vi "Launch Rectangular Mask.vi"(4 "Color":u32, 6 "Transparency":u8, 9 "Monitor":i32, 10 "Bounds":T2) -> (2 "Panels (cluster)":T1, 3 "Panels (array)":refnum<vi>[](array[refnum]))   [LabVIEW 2016, in "Rectangle Mask.lvclass"]
uses:
  Classes/Rectangle Mask/Rectangle Mask.lvclass
  <vilib>/Utility/miscctls.llb/LVRectTypeDef.ctl
  Classes/Rectangle Mask/Panels.ctl
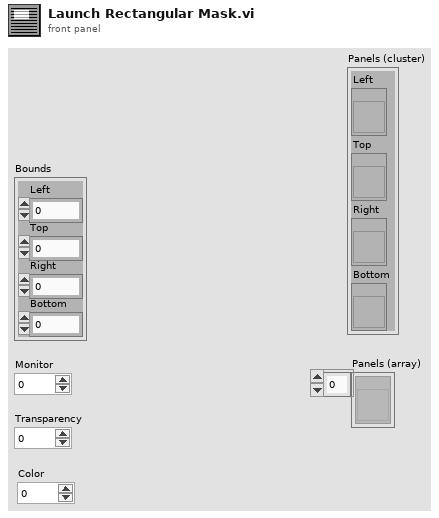
[diagram p1: front panel]
types:
  T1 = typedef "Rectangle Mask.lvclass/Panels.ctl" = cluster{"Left":refnum<vi>, "Top":refnum<vi>, "Right":refnum<vi>, "Bottom":refnum<vi>}
  T2 = typedef "LVRectTypeDef.ctl" = cluster{"Left":i16, "Top":i16, "Right":i16, "Bottom":i16}
  T3 = enum32{"Invalid", "Standard", "Closed", "Hidden", "Minimized", "Maximized"}
  T4 = typedef "LVAllMonitorsDisplayTypeDef.ctl" = cluster{"Bounds":cluster{"Left":i16, "Top":i16, "Right":i16, "Bottom":i16}, "Depth":i16}[]
  T5 = cluster{"Bounds":cluster{"Left":i16, "Top":i16, "Right":i16, "Bottom":i16}, "Depth":i16}
  T6 = cluster{"Left":i16, "Top":i16, "Right":i16, "Bottom":i16}
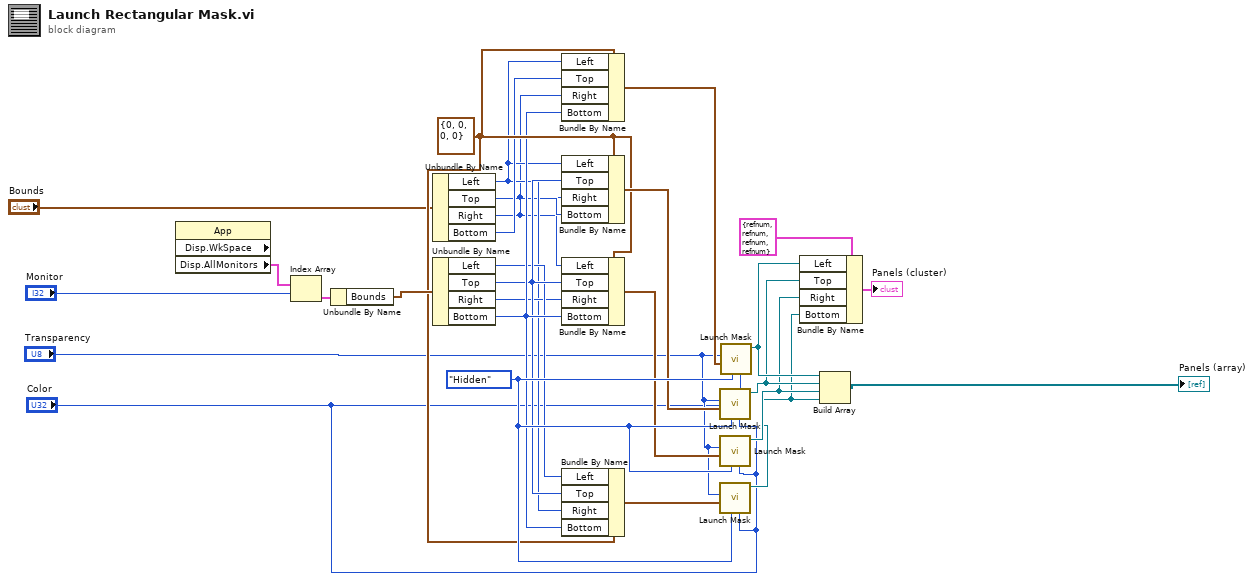
[diagram p0: block diagram]
diagram:
  w24 = T3."Hidden" ("Panel State")
  w20 = T2 {"Left"=0, "Top"=0, "Right"=0, "Bottom"=0} ("Front Panel Window:Panel Bounds")
  n1 = property class="App" props=["Disp.WkSpace", "Disp.AllMonitors"]() -> ("Disp.AllMonitors"=w25:T4)  [unwired: 2 in, 3 out]
  n2 = Index Array(array=w25, index="Monitor") -> (element=w27:T5)
  n3 = Unbundle By Name(w27) -> ("Bounds"=w28:T6)
  n4 = Unbundle By Name("Bounds") -> ("Left"=w14:i16, "Top"=w13:i16, "Right"=w12:i16, "Bottom"=w16:i16)
  n5 = Unbundle By Name(w28) -> ("Left"=w17:i16, "Top"=w18:i16, "Right"=w15:i16, "Bottom"=w19:i16)
  n6 = Bundle By Name(cluster=w20, "Left"=w14, "Top"=w16, "Right"=w12, "Bottom"=w19) -> (w23:T2)
  n7 = Bundle By Name(cluster=w20, "Left"=w14, "Top"=w18, "Right"=w12, "Bottom"=w13) -> (w22:T2)
  n8 = Bundle By Name(cluster=w20, "Left"=w12, "Top"=w18, "Right"=w15, "Bottom"=w19) -> (w21:T2)
  n9 = Bundle By Name(cluster=w20, "Left"=w17, "Top"=w18, "Right"=w14, "Bottom"=w19) -> (w11:T2)
  n10 = call "Launch Mask.vi"("Pane Color"="Color", "Panel State"=w24, "Bounds"=w22, "Panel Transparency"="Transparency") -> ("reference out"=w7:refnum<vi>)  [unwired: 6 in, 1 out]
  n11 = call "Launch Mask.vi"("Pane Color"="Color", "Panel State"=w24, "Bounds"=w21, "Panel Transparency"="Transparency") -> ("reference out"=w6:refnum<vi>)  [unwired: 6 in, 1 out]
  n12 = call "Launch Mask.vi"("Pane Color"="Color", "Panel State"=w24, "Bounds"=w11, "Panel Transparency"="Transparency") -> ("reference out"=w5:refnum<vi>)  [unwired: 6 in, 1 out]
  n13 = call "Launch Mask.vi"("Pane Color"="Color", "Panel State"=w24, "Bounds"=w23, "Panel Transparency"="Transparency") -> ("reference out"=w8:refnum<vi>)  [unwired: 6 in, 1 out]
  n14 = Bundle By Name(cluster=T1 {"Left"=refnum, "Top"=refnum, "Right"=refnum, "Bottom"=refnum} ("Panels Out"), "Left"=w8, "Top"=w7, "Right"=w6, "Bottom"=w5) -> (→"Panels (cluster)":T1)
  n15 = Build Array(w8, w7, w6, w5) -> (→"Panels (array)":refnum<vi>[])
